vi "Set Cursor Icon.vi"(0 "cursor icon":u16, 11 "error in":errorcluster) -> (15 "error out":errorcluster)   [LabVIEW 2021, in "Converter.lvlib"]
uses:
  Converter.lvlib
  <vilib>/Utility/cursorutil.llb/Set Cursor (Icon Pict).vi
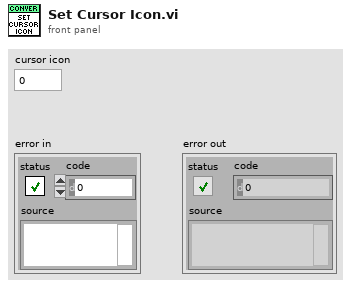
[diagram p1: front panel]
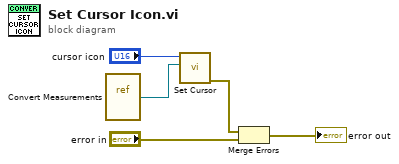
[diagram p0: block diagram]
diagram:
  n1 = vi-ref "Convert Measurements.vi"() -> (w4:refnum<vi>)
  n2 = call-poly <vilib>:"Set Cursor.vi"("VI reference (current VI)"=w4, "icon"="cursor icon") -> ("error out"=w3:errorcluster)  [unwired: 8 in, 1 out]
  n3 = Merge Errors(w3, "error in") -> (→"error out":errorcluster)
